vi "QEcho.vi"(8 "error in (no error)":errorcluster, 11 "VISA resource name":refnum<visa-resource-name>) -> (0 "error out":errorcluster, 2 "output":string, 3 "VISA resource name out":refnum<visa-resource-name>)   [LabVIEW 2013, in "Newport 1830-C.lvlib"]
doc: "0=off\n1=on"
uses:
  Newport 1830-C.lvlib
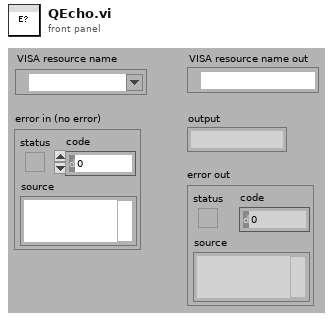
[diagram p1: front panel]
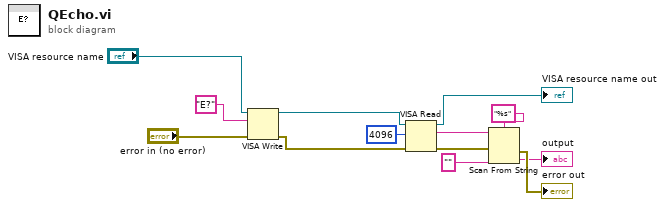
[diagram p0: block diagram]
diagram:
  n1 = VISA Write(VISA resource name="VISA resource name", write buffer="E?" ("command"), error in (no error)="error in (no error)") -> (VISA resource name out=w11:refnum<visa-resource-name>, error out=w10:errorcluster)  [unwired: 1 out]
  n2 = VISA Read(VISA resource name=w11, byte count=u32 4096, error in (no error)=w10) -> (VISA resource name out=→"VISA resource name out":refnum<visa-resource-name>, read buffer=w6:string, error out=w4:errorcluster)  [unwired: 1 out]
  n3 = Scan From String(format string="%s", input string=w6, error in=w4, default 1="" ("default value 1")) -> (error out=→"error out":errorcluster, output 1=→"output":string)  [unwired: 1 in, 2 out]
